vi "LAYER ANALYZE.vi"() -> ()   [LabVIEW 2014]
uses:
  <vilib>/Analysis/NI_AALPro.lvlib
panel:
  out "Load count":i32
  out "A Scan":sgl[](graph)
  out "B Scan":sgl[][](graph)
  in  "LOAD":bool
  in  "stop":bool
  in  "Record length":i32=150
  in  "File path":path=path "D:/Workspace/Giang/Labview/Data/29e79"
  in  "File extension":string=".dat"
  in  "File name":string="29e79"
  in  "Number of B scan":i32=550
  in  "Number of records":i32=1400
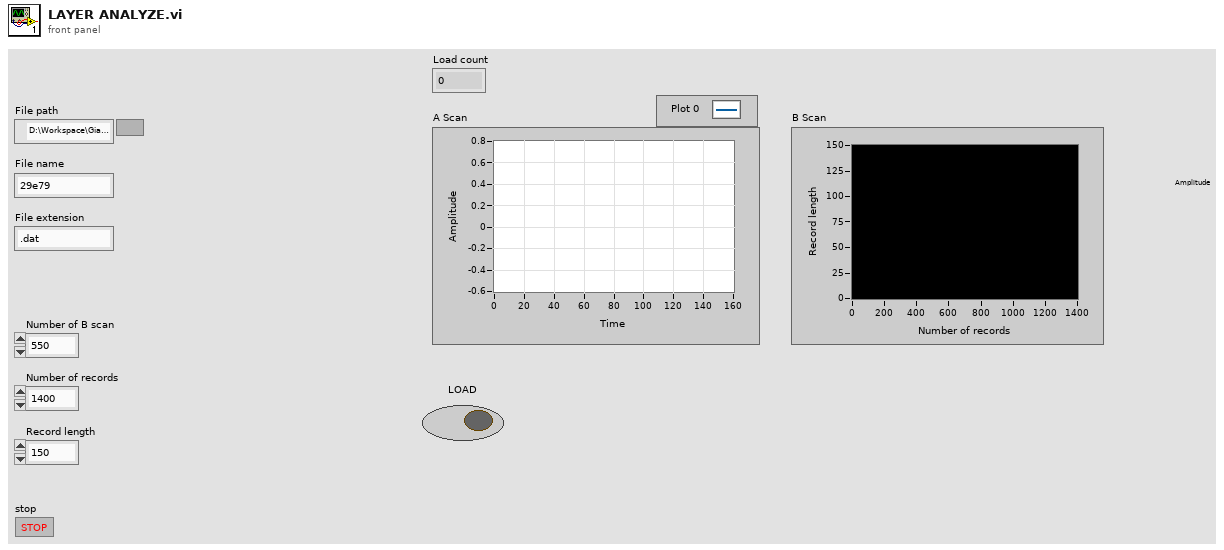
[diagram p1: front panel]
types:
  T1 = enum16{"big-endian, network order", "native, host order", "little-endian"}
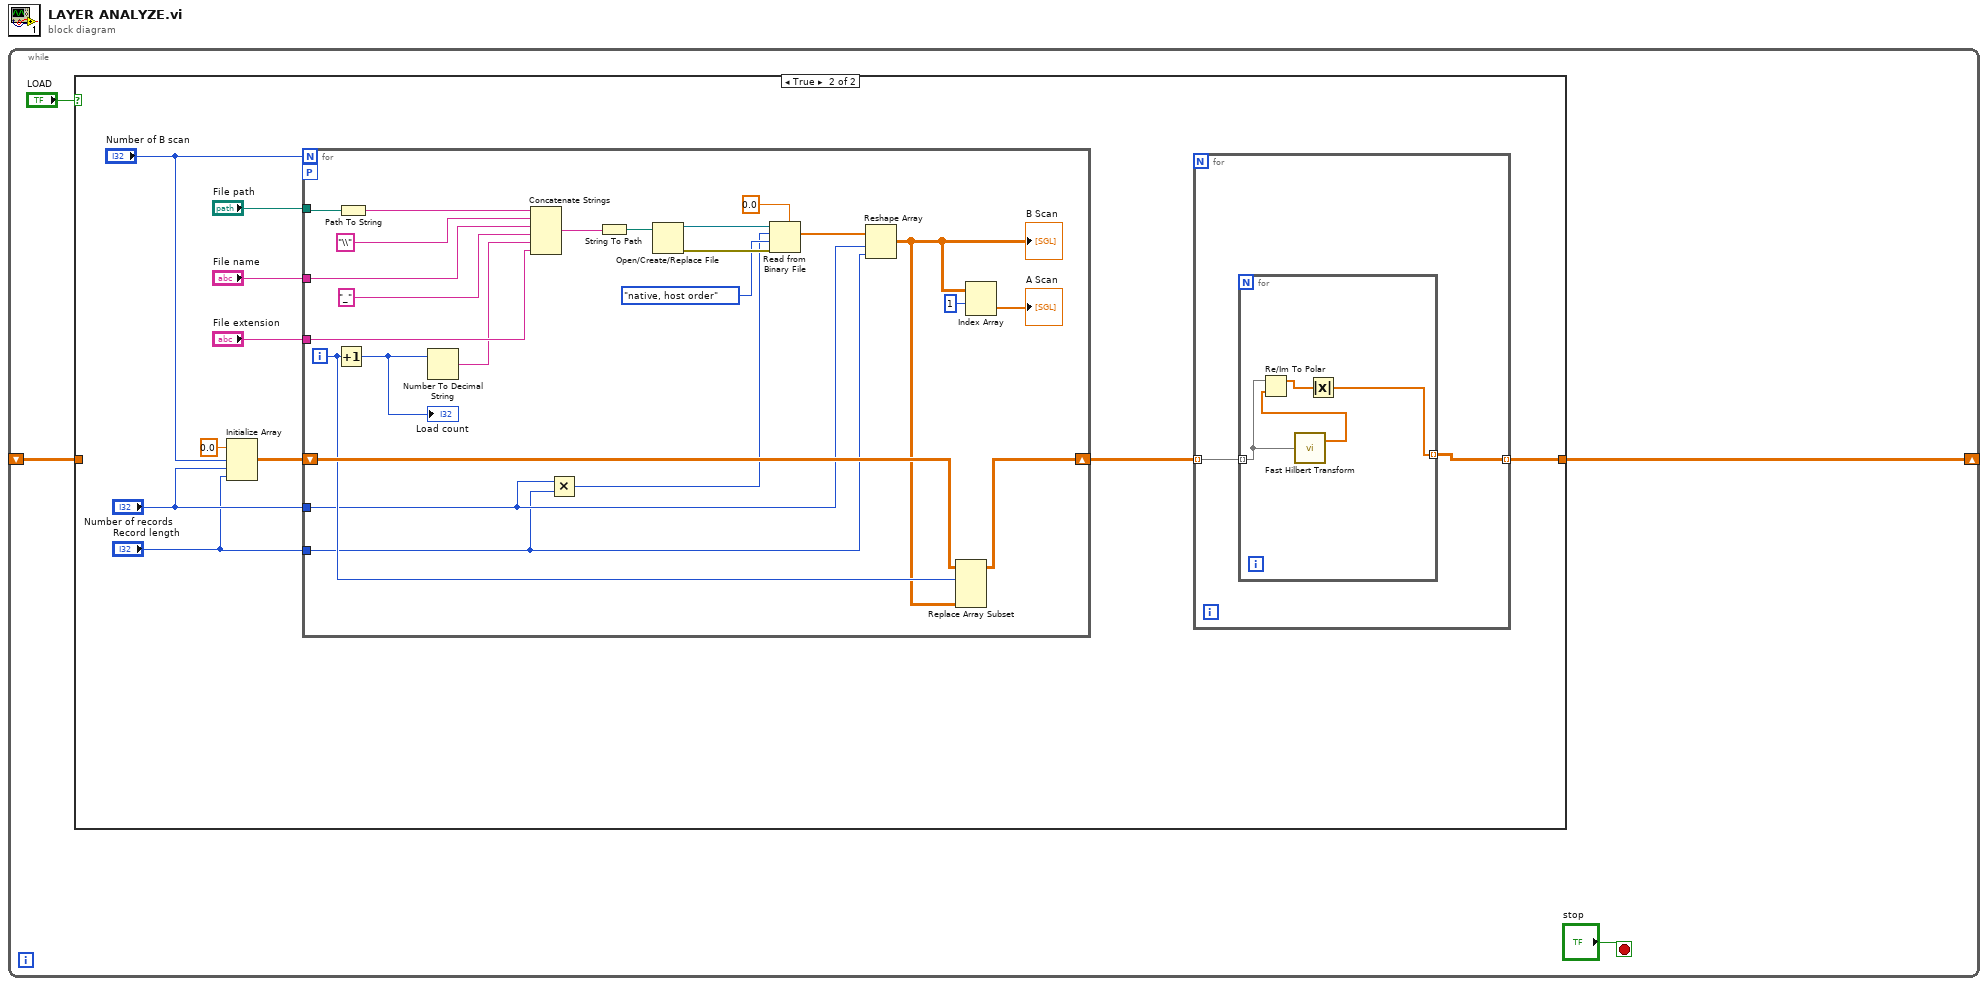
[diagram p0: block diagram]
diagram:
  n1 = while {
    shift-right: [w2] -> _
    shift-left: _ -> [w1]
    stop <- "stop" stop-if-true
    n2 = case shown="True" "LOAD" {
      tunnel: [w5 w7] -> w2
      tunnel: w1 -> [w5 _]
      frame False {
      }
      frame True {
        n3 = Initialize Array(sgl 0.0 ("element"), "Number of B scan", "Number of records", "Record length") -> (w8:sgl[][][])
        n4 = for {
          N: "Number of B scan" -> [_]
          tunnel: "File path" -> [w29]
          tunnel: "File name" -> [w33]
          tunnel: "File extension" -> [w32]
          tunnel: "Number of records" -> [w24]
          tunnel: "Record length" -> [w23]
          shift-right: [w26] -> w6
          shift-left: w8 -> [w28]
          workers-P: _ -> [_]
          i -> [w27]
          n5 = Increment(x=w27) -> (x+1=w31:i32)
          "Load count" <- w31
          n6 = Path To String(path=w29) -> (string=w34:string)
          n7 = Number To Decimal String(number=w31) -> (decimal integer string=w30:string)  [unwired: 1 in]
          n8 = Concatenate Strings(w34, "\\" ("string"), w33, "_" ("string"), w30, w32) -> (w37:string)
          n9 = Multiply(x=w24, y=w23) -> (x*y=w22:i32)
          n10 = String To Path(string=w37) -> (path=w38:path)
          n11 = Open/Create/Replace File(file path (use dialog)=w38) -> (refnum out=w39:refnum<file>, error out=w41:errorcluster)  [unwired: 5 in, 1 out]
          n12 = Read from Binary File(5:sgl 0.0, 8:w41, 9:T1."native, host order" ("byte order (0:big-endian, network order)"), 10:w22, 11:w39) -> (2:w42:sgl[])  [unwired: 1 in, 3 out]
          n13 = Reshape Array(w42, w24, w23) -> (w25:sgl[][])
          "B Scan" <- w25
          n14 = Replace Array Subset(array=w28, new element=w25, index (dim 0)=w27) -> (w26:sgl[][][])  [unwired: 2 in]
          n15 = Index Array(array=w25, index (row)=1) -> (element=→"A Scan":sgl[])  [unwired: 1 in]
        }
        n16 = for {
          tunnel: [w17] -> w7 mode=indexing
          tunnel: w6 -> [w16] mode=indexing
          n17 = for {
            tunnel: [w18] -> w17 mode=indexing
            tunnel: w16 -> [w21] mode=indexing
            n18 = call <vilib>:"Fast Hilbert Transform.vi"("X"=w21) -> ("Hilbert{X}"=w20:dbl[])  [unwired: 1 out]
            n19 = Re/Im To Polar(2:w20, 3:w21) -> (1:w19:dbl[])  [unwired: 1 out]
            n20 = Absolute Value(x=w19) -> (abs(x)=w18:dbl[])
          }
        }
      }
    }
  }
